vi "SQLRowCount.vi"(4 "error in (no error)":errorcluster, 7 "InputHandle":i32) -> (0 "error out":errorcluster, 2 "RowCount":i32, 3 "OutputHandle":i32)   [LabVIEW 2011]
doc: "Donne le nombre de lignes modifiées par la requête"
uses:
  Odbc32.dll
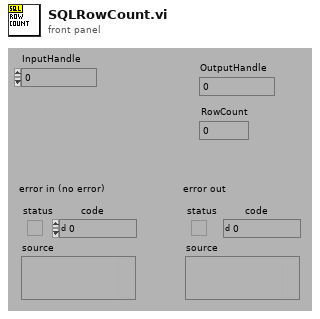
[diagram p1: front panel]
types:
  T1 = enum16{"NOPE", "SQL_HANDLE_ENV", "SQL_HANDLE_DBC", "SQL_HANDLE_STMT", "SQL_HANDLE_DESC"}
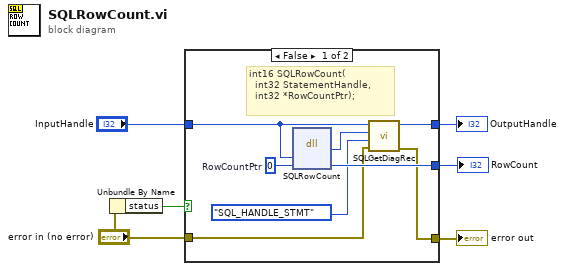
[diagram p0: block diagram]
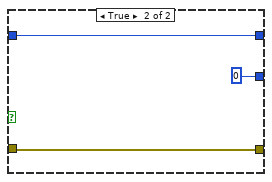
[diagram p2: hidden frame]
diagram:
  n1 = Unbundle By Name("error in (no error)") -> ("status"=w1:bool)
  n2 = case shown="False" w1 {
    tunnel: [w14 0] -> w6
    tunnel: [w12 w16] -> w5
    tunnel: "InputHandle" -> [w11 w16]
    tunnel: [w9 w15] -> w3
    tunnel: "error in (no error)" -> [w8 w15]
    frame False {
      w13 = 0  # RowCountPtr
      # "int16 SQLRowCount(\n  int32 StatementHandle, \n  int32 *RowCountPtr);"
      n3 = dll-call lib="Odbc32.dll" fn="SQLRowCount"("StatementHandle"=w11, "RowCountPtr"=w13) -> (w10:i16, "RowCountPtr"=w14:i32)  [unwired: 4 in, 2 out]
      n4 = call "SQLGetDiagRec.vi"("error in (no error)"=w8, "HandleType"=T1."SQL_HANDLE_STMT", "Status (SQL_SUCCESS=0)"=w10, "Input Handle"=w11) -> ("error out"=w9:errorcluster, "Output Handle"=w12:i32)  [unwired: 2 out]
    }
    frame True {
    }
  }
  "RowCount" <- w6
  "OutputHandle" <- w5
  "error out" <- w3
